vi "Stop Do.vi"(8 "error in":errorcluster, 11 "Task Actor in":refnum<class "Task Actor.lvclass">) -> (0 "error out":errorcluster, 3 "Task Actor out":refnum<class "Task Actor.lvclass">)   [LabVIEW 2023, in "Task Actor.lvlib" / "Task Actor.lvclass"]
uses:
  Task Actor.lvclass
  <vilib>/ActorFramework/Actor/Actor.lvclass/Actor.ctl
  Task Actor.lvclass/Task Actor.ctl
  Task Base/Task Base.lvclass
  <vilib>/ActorFramework/Actor/Actor.lvclass
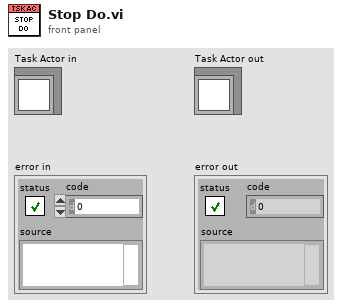
[diagram p1: front panel]
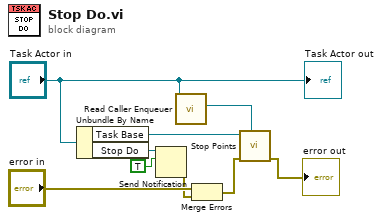
[diagram p0: block diagram]
diagram:
  n1 = Unbundle By Name("Task Actor in") -> ("Task Base"=w4:refnum<class "Task Base.lvclass">, "Stop Do"=w9:refnum<notifier>)
  n2 = Send Notification(notification=TRUE, notifier=w9) -> (error out=w3:errorcluster)  [unwired: 1 in, 1 out]
  n3 = call <vilib>:"Read Caller Enqueuer.vi"("Actor"="Task Actor in") -> ("Caller Enqueuer"=w2:refnum<class "Message Enqueuer.lvclass">)  [unwired: 10 in]
  n4 = Merge Errors("error in", w3) -> (w6:errorcluster)
  n5 = call-dynamic "Stop Points.vi"("Series Enqueuer"=w2, "error in"=w6, "Task Base in"=w4) -> ("error out"=→"error out":errorcluster)  [unwired: 7 in, 1 out]
  "Task Actor out" <- "Task Actor in"
